vi "Get Measurement Details.vi"(8 "error in":errorcluster) -> (0 "error out":errorcluster, 1 "measurement annotations":T1[](array[typedef]), 2 "service class":string, 3 "measurement details":T2)   [LabVIEW 2021, in "Multi-Channel Output Voltage Accuracy_PMIC.lvlib"]
uses:
  Multi-Channel Output Voltage Accuracy_PMIC.lvlib
  <vilib>/Plug-In SDKs/Measurements/Helpers/TypeDefs/Measurement Details.ctl
  <vilib>/Plug-In SDKs/Measurements/Helpers/TypeDefs/Measurement Annotation.ctl
  <vilib>/Plug-In SDKs/Measurements/NI Measurement Plug-In SDK.lvlib
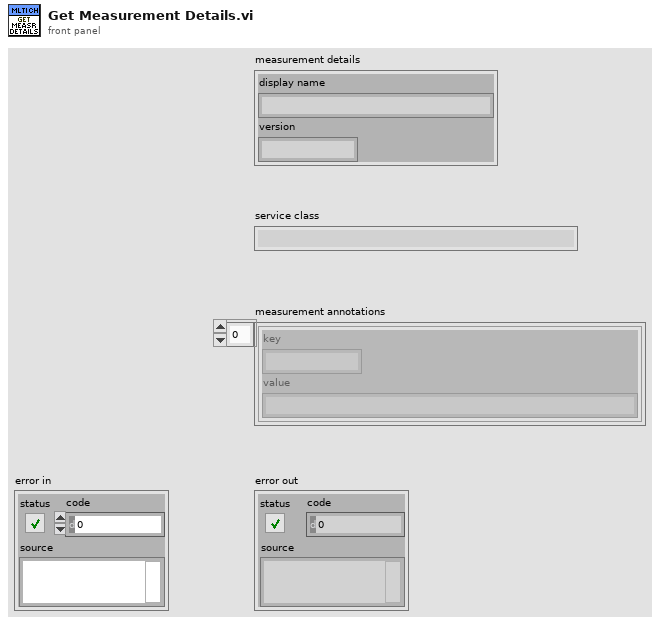
[diagram p1: front panel]
types:
  T1 = typedef "NI Measurement Plug-In SDK.lvlib/Measurement Annotation.ctl" = cluster{"key":string, "value":string}
  T2 = typedef "NI Measurement Plug-In SDK.lvlib/Measurement Details.ctl" = cluster{"display name":string, "version":string}
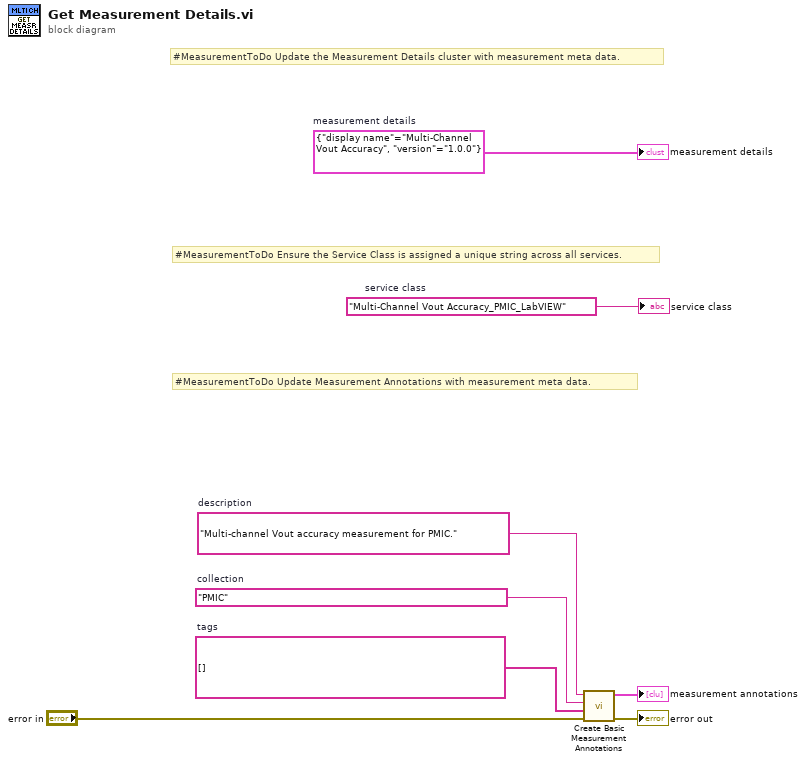
[diagram p0: block diagram]
diagram:
  w1 = string[] []  # tags
  w2 = "PMIC"  # collection
  w3 = "Multi-channel Vout accuracy measurement for PMIC."  # description
  w7 = T2 {"display name"="Multi-Channel Vout Accuracy", "version"="1.0.0"}  # measurement details
  w8 = "Multi-Channel Vout Accuracy_PMIC_LabVIEW"  # service class
  # "#MeasurementToDo Update Measurement Annotations with measurement meta data."
  # "#MeasurementToDo Ensure the Service Class is assigned a unique string across all services."
  # "#MeasurementToDo Update the Measurement Details cluster with measurement meta data."
  n1 = call <vilib>:"Create Basic Measurement Annotations.vi"("error in"="error in", "tags"=w1, "collection"=w2, "description"=w3) -> ("error out"=→"error out":errorcluster, "measurement annotations"=→"measurement annotations":T1[])  [unwired: 6 in]
  "measurement details" <- w7
  "service class" <- w8
